vi "Set Vector Magnitude.vi"(8 "error in":errorcluster, 10 "Manitude":dbl, 11 "PVector in":refnum<class "PVector.lvclass">) -> (0 "error out":errorcluster, 3 "PVector out":refnum<class "PVector.lvclass">)   [LabVIEW 2016, in "PVector.lvclass"]
doc: "Set vector <B>V</B> magnitude ||<B>V</B>|| while preserving its direction."
uses:
  PVector.lvclass
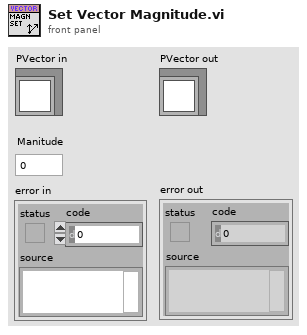
[diagram p1: front panel]
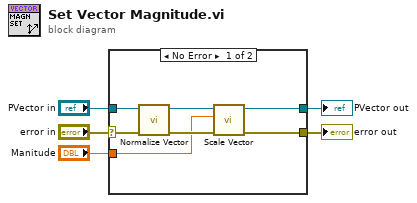
[diagram p0: block diagram]
diagram:
  n1 = case shown="No Error" "error in" {
    selector: "error in" -> [w11 w14]
    tunnel: [w6 w14] -> w4
    tunnel: [w7 w13] -> w2
    tunnel: "PVector in" -> [w12 w13]
    tunnel: "Manitude" -> [w8 _]
    frame No Error {
      n2 = call "Normalize Vector.vi"("error in"=w11, "PVector in"=w12) -> ("error out"=w9:errorcluster, "norm(PVector) out"=w10:refnum<class "PVector.lvclass">)  [unwired: 8 in]
      n3 = call "Scale Vector.vi"("error in"=w9, "n (1)"=w8, "PVector V"=w10) -> ("error out"=w6:errorcluster, "PVector nV"=w7:refnum<class "PVector.lvclass">)  [unwired: 7 in]
    }
    frame Error {
    }
  }
  "error out" <- w4
  "PVector out" <- w2
